vi "VIsionCode2.vi"(7 "error in":errorcluster) -> (27 "error out":errorcluster)   [LabVIEW 2011]
uses:
  <vilib>/vision/NI_Vision_Development_Module.lvlib
panel:
  out "Image Out":T1(plugin-control)
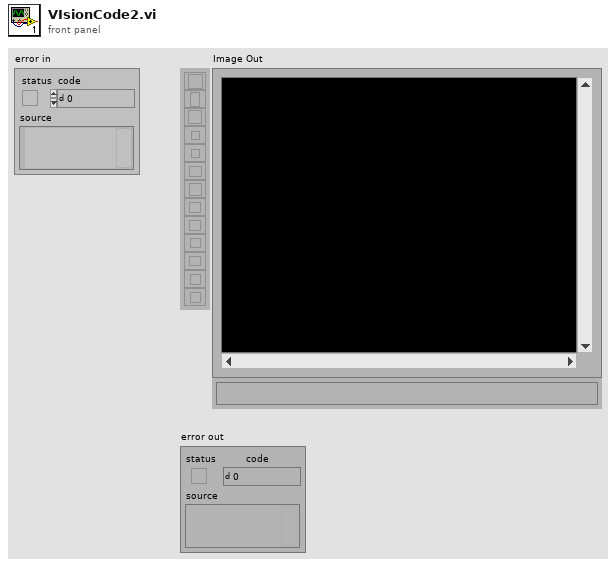
[diagram p1: front panel]
types:
  T1 = typedef "IMAQ Image.ctl" = refnum<image>
  T2 = cluster{"ID":enum32{"External", "Internal"}, "Type":u32, "Coordinates":i32[]}[]
  T3 = enum16{"Get First Edge", "Get First + Last Edge", "Get All Edges"}
  T4 = cluster{"Level Type":enum32{"Absolute Value", "Relative value"}, "Threshold Level":i32, "Hysteresis":i32}
  T5 = cluster{"Measurement Parameter":i32, "Range Lower Value":dbl, "Range Upper Value":dbl, "Range":bool, "Measurement Type":bool}[]
  T6 = typedef "Image Type" = u32
  T7 = cluster{"Global Rectangle":i32[], "Contours":cluster{"ID":enum32{"External", "Internal"}, "Type":u32, "Coordinates":i32[]}[]}
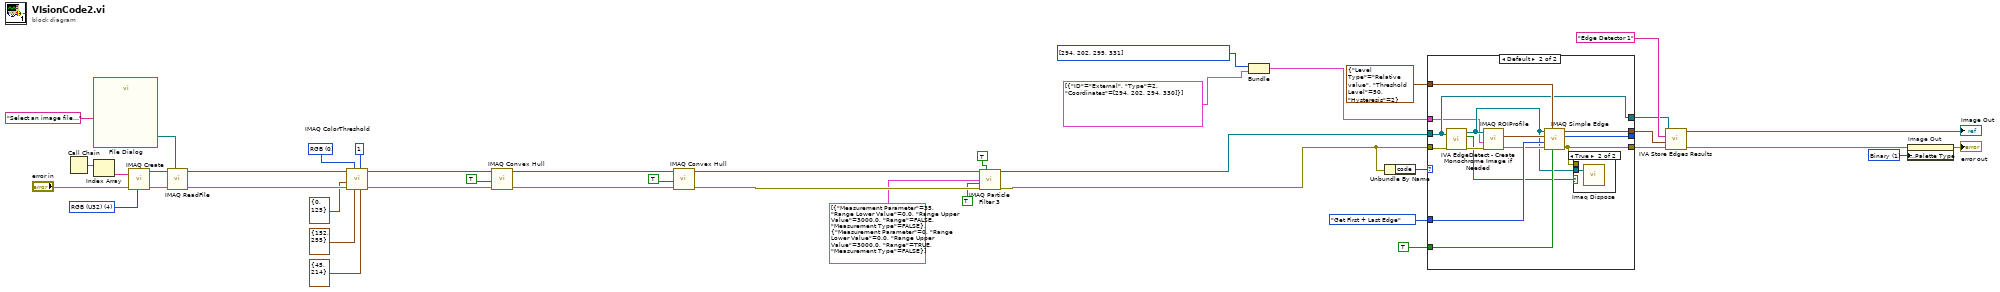
[diagram p0: block diagram]
diagram:
  w5 = u32 1 items=["Grayscale", "Binary", "Gradient", "Rainbow", "Temperature", "User Defined"] ("Palette")
  w33 = u16 0 items=["RGB", "HSL", "HSV", "HSI"] ("Color Mode")
  w35 = T6 4 items=["Grayscale (U8)", "Grayscale (I16)", "Grayscale (SGL)", "Complex (CSG)", "RGB (U32)", "HSL (U32)", "RGB (U64)", "Grayscale (U16)"] ("Image Type")
  n1 = Call Chain() -> (call chain=w39:string[])
  n2 = Index Array(array=w39) -> (element=w38:string)  [unwired: 1 in]
  n3 = call "File Dialog"("prompt"="Select an image file...") -> ("selected path"=w36:path)  [unwired: 6 in, 8 out]
  n4 = call "IMAQ Create"("Image Name"=w38, "Image Type"=w35, "error in (no error)"="error in") -> ("New Image"=w42:T1, "error out"=w41:errorcluster)  [unwired: 1 in, 1 out]
  n5 = call "IMAQ ReadFile"("File Path"=w36, "error in (no error)"=w41, "Image"=w42) -> ("error out"=w43:errorcluster, "Image Out"=w29:T1)  [unwired: 2 in, 5 out]
  n6 = call "IMAQ ColorThreshold"("Blue or Luma or Val or Inten Range"=cluster{"Lower value":i32, "Upper value":i32} {"Lower value"=45, "Upper value"=214}, "Replace Value"=1, "Green or Sat Range"=cluster{"Lower value":i32, "Upper value":i32} {"Lower value"=152, "Upper value"=255}, "Color Mode"=w33, "error in (no error)"=w43, "Red or Hue Range"=cluster{"Lower value":i32, "Upper value":i32} {"Lower value"=0, "Upper value"=125}, "Image Src"=w29) -> ("error out"=w28:errorcluster, "Image Dst Out"=w27:T1)  [unwired: 1 in, 2 out]
  n7 = call "IMAQ Convex Hull"("error in (no error)"=w28, "Connectivity 4/8 (8)"=TRUE, "Image Src"=w27) -> ("error out"=w25:errorcluster, "Image Dst Out"=w24:T1)  [unwired: 1 in, 6 out]
  n8 = call "IMAQ Convex Hull"("error in (no error)"=w25, "Connectivity 4/8 (8)"=TRUE, "Image Src"=w24) -> ("error out"=w22:errorcluster, "Image Dst Out"=w18:T1)  [unwired: 1 in, 6 out]
  n9 = call "IMAQ Particle Filter 3"("Image Src"=w18, "Connectivity 4/8 (8)"=TRUE, "Selection Values"=T5 [{"Measurement Parameter"=35, "Range Lower Value"=0.0, "Range Upper Value"=3000.0, "Range"=FALSE, "Measurement Type"=FALSE}, {"Measurement Parameter"=0, "Range Lower Value"=0.0, "Range Upper Value"=3000.0, "Range"=TRUE, "Measurement Type"=FALSE}], "Keep/Remove Particles (F)"=TRUE ("Keep/Remove Particles"), "error in (no error)"=w22) -> ("Image Dst Out"=w14:T1, "error out"=w19:errorcluster)  [unwired: 4 in, 5 out]
  n10 = Bundle("Global Rectangle"=i32[] [294, 202, 295, 331], "Contours"=T2 [{"ID"=enum."External", "Type"=2, "Coordinates"=[294, 202, 294, 330]}]) -> (w1:T7)  [unwired: 1 in]
  n11 = Unbundle By Name(w19) -> ("code"=w9:i32)
  n12 = case shown="Default" w9 {
    tunnel: T4 {"Level Type"=enum."Relative value", "Threshold Level"=50, "Hysteresis"=2} ("Threshold Parameters") -> [_ w58]
    tunnel: T3."Get First + Last Edge" ("Process") -> [_ w57]
    tunnel: [_ w56] -> _
    tunnel: w19 -> [_ w50]
    tunnel: w14 -> [w44 w51]
    tunnel: [_ w53] -> w12
    tunnel: [_ w46] -> w11
    tunnel: TRUE ("Sub-Pixel Accuracy") -> [_ w52]
    tunnel: [w44 w51] -> w7
    tunnel: w1 -> [_ w45]
    frame -1074396199, -1074396198 {
      # "Discard Coordinate System Error"
    }
    frame Default {
      n13 = call <vilib>:"IVA EdgeDetect - Create Monochrome Image if Needed.vi"("error in (no error)"=w50, "Image In"=w51) -> ("error out"=w49:errorcluster, "Mono Image Created"=w47:bool, "Mono Image Out"=w48:T1)  [unwired: 7 out]
      n14 = call "IMAQ ROIProfile"("error in (no error)"=w49, "ROI Descriptor"=w45, "Image"=w48) -> ("error out"=w54:errorcluster, "Pixel Coordinates"=w55:cluster{"X":u32, "Y":u32}[])  [unwired: 4 out]
      n15 = call "IMAQ Simple Edge"("Sub-Pixel Accuracy"=w52, "Threshold Parameters"=w58, "error in (no error)"=w54, "Process"=w57, "Pixel Coordinates"=w55, "Image Src"=w48) -> ("error out"=w46:errorcluster, "Number of Edges"=w56:i32, "Edges Coordinates"=w53:cluster{"X":sgl, "Y":sgl}[])  [unwired: 3 out]
      n16 = case shown="True" w47 {
        tunnel: w48 -> [_ w59]
        tunnel: w46 -> [_ _]
        frame False {
        }
        frame True {
          n17 = call "Imaq Dispose"("Image"=w59) -> ()  [unwired: 2 in, 4 out]
        }
      }
    }
  }
  n18 = call <vilib>:"IVA Store Edges Results.vi"("error in (no error)"=w11, "Edge Coordinates"=w12, "Step Name"="Edge Detector 1", "Image in"=w7) -> ("error out"=w10:errorcluster, "Image dup"=→"Image Out":T1)  [unwired: 6 out]
  n19 = property on="Image Out" class="ImageControl"(error in=w10, "Palette:Palette Type"=w5) -> (error out=→"error out":errorcluster)  [unwired: 1 in, 1 out]
